vi "InitBrd.vi"(0 "xckdly":u32 format="%.0x", 3 "board_sel":u32=1 format="%.0x", 4 "pixel":u32=5400, 5 "flag816":u32=1) -> ()   [LabVIEW 2015]
uses:
  ESLSCDLL.dll
panel:
  in  "pclk":u32 format="%.0x"
  # "set read frequency"
  # "8bit=2/12-16bit=1"
  # "not used"
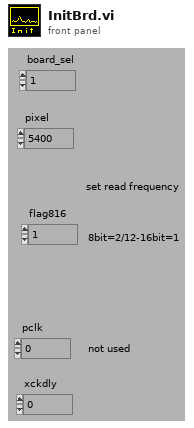
[diagram p1: front panel]
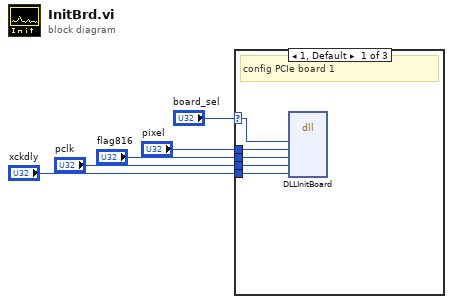
[diagram p0: block diagram]
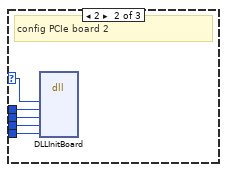
[diagram p2: hidden frame]
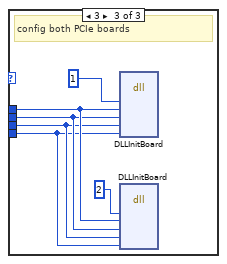
[diagram p3: hidden frame]
diagram:
  n1 = case shown="1, Default" "board_sel" {
    selector: "board_sel" -> [w10 w11 _]
    tunnel: "pixel" -> [w9 w12 w19]
    tunnel: "flag816" -> [w8 w13 w18]
    tunnel: "pclk" -> [w7 w14 w17]
    tunnel: "xckdly" -> [w6 w15 w16]
    frame 1, Default {
      # "config PCIe board 1"
      n2 = dll-call lib="C:/ENTW/PCIE/lv64/board.vis/ESLSCDLL.dll" fn="DLLInitBoard"("drv"=w10, "pixel"=w9, "flag816"=w8, "pclk"=w7, "xckdelay"=w6) -> ()  [unwired: 9 in, 2 out]
    }
    frame 2 {
      # "config PCIe board 2"
      n3 = dll-call lib="C:/ENTW/PCIE/lv64/board.vis/ESLSCDLL.dll" fn="DLLInitBoard"("drv"=w11, "pixel"=w12, "flag816"=w13, "pclk"=w14, "xckdelay"=w15) -> ()  [unwired: 9 in, 2 out]
    }
    frame 3 {
      # "config both PCIe boards"
      n4 = dll-call lib="C:/ENTW/PCIE/lv64/board.vis/ESLSCDLL.dll" fn="DLLInitBoard"("drv"=u32 1, "pixel"=w19, "flag816"=w18, "pclk"=w17, "xckdelay"=w16) -> ()  [unwired: 9 in, 2 out]
      n5 = dll-call lib="C:/ENTW/PCIE/lv64/board.vis/ESLSCDLL.dll" fn="DLLInitBoard"("drv"=u32 2, "pixel"=w19, "flag816"=w18, "pclk"=w17, "xckdelay"=w16) -> ()  [unwired: 9 in, 2 out]
    }
  }
